vi "Move Non LabVIEW Files.vi"(8 "Error In":errorcluster, 11 "Revert Config":T1={"Revert Paths"={"Archive Path"=path "D:/workspace/revert/todo/todo.zip", "Unzip Directory"=path "D:/workspace/revert/unzip", "Backsave Directory"=path "D:/workspace/revert/backsave", "Output Archive"=path "D:/workspace/revert/output/out.zip", "Backsave Common Directory"=path "D:/workspace/revert/backsave"}, "LabVIEW Files"={"Projects"=[], "Libraries"=[], "Classes"=[], "XControls"=[], "VIs and Controls"=[], "Non LV Files"=[]}, "LabVIEW Version"=enum."8.0"}) -> (0 "Error Out":errorcluster, 3 "Revert Config":T1={"Revert Paths"={"Archive Path"=path "D:/workspace/revert/todo/todo.zip", "Unzip Directory"=path "D:/workspace/revert/unzip", "Backsave Directory"=path "D:/workspace/revert/backsave", "Output Archive"=path "D:/workspace/revert/output/out.zip", "Backsave Common Directory"=path "D:/workspace/revert/backsave"}, "LabVIEW Files"={"Projects"=[], "Libraries"=[], "Classes"=[], "XControls"=[], "VIs and Controls"=[], "Non LV Files"=[]}, "LabVIEW Version"=enum."8.0"})   [LabVIEW 2013, in "LVH-Revert.lvlib"]
uses:
  <vilib>/LabVIEW Hacker/Revert/LVH-Revert.lvlib
  <vilib>/LabVIEW Hacker/Revert/Type Defs/Revert Config.ctl
  <vilib>/LabVIEW Hacker/Revert/Type Defs/Paths.ctl
  <vilib>/LabVIEW Hacker/Revert/Type Defs/LabVIEW Files.ctl
  <vilib>/LabVIEW Hacker/LVH-Toolbox/Common/Private/Type Defs/LabVIEW Version.ctl
  <vilib>/LabVIEW Hacker/LVH-Toolbox/Common/LVH-Common.lvlib
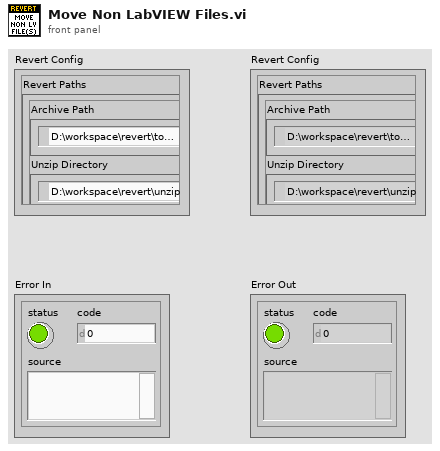
[diagram p1: front panel]
types:
  T1 = typedef "LVH-Revert.lvlib/Revert Config.ctl" = cluster{"Revert Paths":T2, "LabVIEW Files":T3, "LabVIEW Version":T4}
  T2 = typedef "LVH-Revert.lvlib/Paths.ctl" = cluster{"Archive Path":path, "Unzip Directory":path, "Backsave Directory":path, "Output Archive":path, "Backsave Common Directory":path}
  T3 = typedef "LVH-Revert.lvlib/LabVIEW Files.ctl" = cluster{"Projects":path[], "Libraries":path[], "Classes":path[], "XControls":path[], "VIs and Controls":path[], "Non LV Files":path[]}
  T4 = typedef "LVH-Toolbox.lvlib/LVH-Common.lvlib/LabVIEW Version.ctl" = enum16{"8.0", "8.2", "8.6", "9.0", "10.0", "11.0", "12.0", "13.0"}
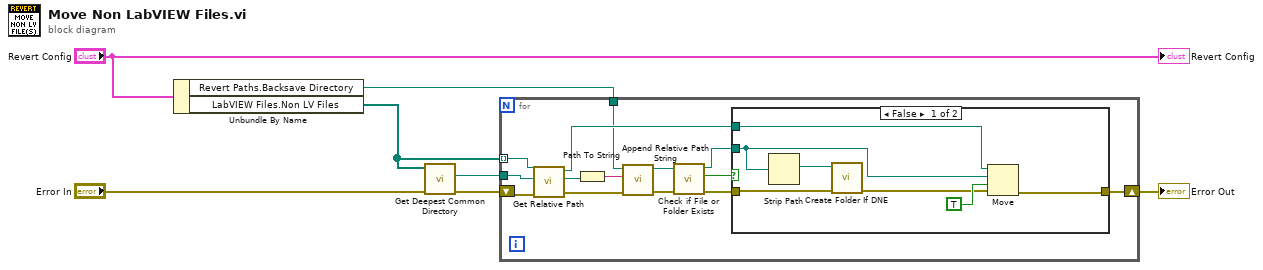
[diagram p0: block diagram]
diagram:
  n1 = Unbundle By Name("Revert Config") -> ("Revert Paths.Backsave Directory"=w1:path, "LabVIEW Files.Non LV Files"=w2:path[])
  n2 = call <vilib>:"Get Deepest Common Directory.vi"("Error In"="Error In", "File Paths"=w2) -> ("Error Out"=w7:errorcluster, "Deepest Common Path"=w6:path)  [unwired: 7 in, 1 out]
  n3 = for {
    shift-right: [w11] -> w3
    shift-left: w7 -> [w21]
    tunnel: w6 -> [w10]
    tunnel: w2 -> [w9] mode=indexing
    tunnel: w1 -> [w8]
    n4 = call <vilib>:"Get Relative Path.vi"("Error In"=w21, "Relative Path Root"=w10, "File / Folder"=w9) -> ("Error Out"=w18:errorcluster, "Relative Path"=w20:path, "Duplicate File / Folder"=w13:path)  [unwired: 6 in]
    n5 = Path To String(path=w20) -> (string=w19:string)
    n6 = call <vilib>:"Append Relative Path String.vi"("Error In"=w18, "Relative Path"=w19, "Base Path"=w8) -> ("Error Out"=w16:errorcluster, "Absolute Path"=w17:path)  [unwired: 7 in]
    n7 = call <vilib>:"Check if File or Folder Exists.vi"("error in (no error)"=w16, "path"=w17) -> ("error out"=w14:errorcluster, "file or folder exists?"=w15:bool, "dup path"=w12:path)  [unwired: 7 in]
    n8 = case shown="False" w15 {
      tunnel: w14 -> [w25 w29]
      tunnel: w13 -> [w27 _]
      tunnel: w12 -> [w23 _]
      tunnel: [w28 w29] -> w11
      frame False {
        n9 = Strip Path(path=w23) -> (stripped path=w22:path)  [unwired: 1 out]
        n10 = call <vilib>:"Create Folder If DNE.vi"("Error In"=w25, "Folder Path"=w22) -> ("Error Out"=w24:errorcluster)  [unwired: 8 in, 1 out]
        n11 = Move(source path=w27, error in=w24, 9:TRUE ("overwrite (F)"), 10:w23) -> (error out=w28:errorcluster)  [unwired: 1 in, 2 out]
      }
      frame True {
        # "File Exists In Backsave.  Ignore"
      }
    }
  }
  "Error Out" <- w3
  "Revert Config" <- "Revert Config"
